vi "CRYRead structure name.vi"(11 "Flat data structure":string) -> (0 "Curve name":string, 1 "Dimensions":u8, 2 "Version":u16, 3 "Data type":string)   [LabVIEW 2013]
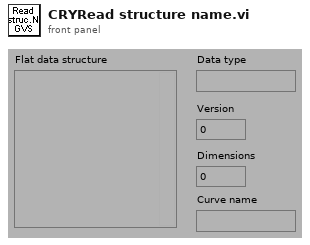
[diagram p1: front panel]
types:
  T1 = cluster{"unsigned byte array[0]":u8, "unsigned byte array[1]":u8, "unsigned byte array[2]":u8}
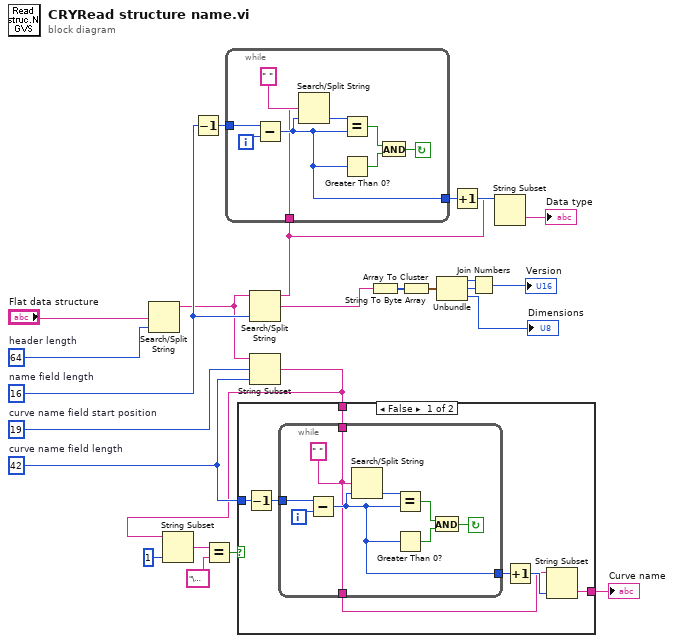
[diagram p0: block diagram]
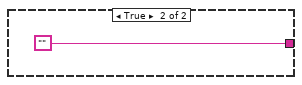
[diagram p2: hidden frame]
diagram:
  w8 = 19  # curve name field start position
  w9 = 42  # curve name field length
  w10 = 16  # name field length
  w18 = 64  # header length
  n1 = Search/Split String(string="Flat data structure", offset (0)=w18) -> (substring before match=w7:string)  [unwired: 3 out]
  n2 = Decrement(x=w10) -> (x-1=w15:i32)
  n3 = Search/Split String(string=w7, offset (0)=w10) -> (substring before match=w12:string, match + rest of string=w20:string)  [unwired: 2 out]
  n4 = while {
    tunnel: w12 -> [w25]
    tunnel: [w26] -> w14
    tunnel: w15 -> [w32]
    i -> [w31]
    stop <- w27 continue-if-true
    n5 = Subtract(x=w32, y=w31) -> (x-y=w26:i32)
    n6 = Search/Split String(string=w25, search string/char (-)=" ", offset (0)=w26) -> (offset of match=w30:i32)  [unwired: 2 out]
    n7 = Equal?(x=w30, y=w26) -> (x = y?=w29:bool)
    n8 = Greater Than 0?(x=w26) -> (x > 0?=w28:bool)
    n9 = And(x=w29, y=w28) -> (x .and. y?=w27:bool)
  }
  n10 = String Subset(string=w7, offset (0)=w8, length (rest)=w9) -> (substring=w1:string)
  n11 = String Subset(string=w1, length (rest)=1 ("length")) -> (substring=w4:string)  [unwired: 1 out]
  n12 = Equal?(x=w4, y="\u0000") -> (x = y?=w2:bool)
  n13 = case shown="False" w2 {
    tunnel: [w40 ""] -> w6
    tunnel: w1 -> [w38 _]
    tunnel: w9 -> [w37 _]
    frame False {
      n14 = Decrement(x=w37) -> (x-1=w36:i32)
      n15 = while {
        tunnel: w38 -> [w41]
        tunnel: [w41] -> w34
        tunnel: [w42] -> w35
        tunnel: w36 -> [w48]
        i -> [w47]
        stop <- w43 continue-if-true
        n16 = Subtract(x=w48, y=w47) -> (x-y=w42:i32)
        n17 = Search/Split String(string=w41, search string/char (-)=" ", offset (0)=w42) -> (offset of match=w46:i32)  [unwired: 2 out]
        n18 = Equal?(x=w46, y=w42) -> (x = y?=w45:bool)
        n19 = Greater Than 0?(x=w42) -> (x > 0?=w44:bool)
        n20 = And(x=w45, y=w44) -> (x .and. y?=w43:bool)
      }
      n21 = Increment(x=w35) -> (x+1=w39:i32)
      n22 = String Subset(string=w34, length (rest)=w39) -> (substring=w40:string)  [unwired: 1 out]
    }
    frame True {
    }
  }
  "Curve name" <- w6
  n23 = String To Byte Array(string=w20) -> (unsigned byte array=w24:u8[])
  n24 = Array To Cluster(array=w24) -> (cluster=w23:T1)
  n25 = Unbundle(w23) -> ("unsigned byte array[0]"=w22:u8, "unsigned byte array[1]"=w21:u8, "unsigned byte array[2]"=→"Dimensions":u8)
  n26 = Increment(x=w14) -> (x+1=w13:i32)
  n27 = Join Numbers(hi=w22, lo=w21) -> ((hi.lo)=→"Version":u16)
  n28 = String Subset(string=w12, length (rest)=w13) -> (substring=→"Data type":string)  [unwired: 1 out]
